vi "Resize Panel to Pane.vi"(8 "error in (no error)":errorcluster, 11 "ActorAutoRegPanel In":refnum<class "ActorAutoRegPanel.lvclass">) -> (0 "error out":errorcluster, 3 "ActorAutoRegPanel Out":refnum<class "ActorAutoRegPanel.lvclass">)   [LabVIEW 2015, in "TestViewables.lvlib" / "ActorAutoRegPanel.lvclass"]
doc: "<License>\nCopyright © 2017 Composed Systems, LLC | All rights reserved\nwww.composed.io\n\nAuthor: Ethan Stern <ethan.stern@composed.io>\n\nThis software is provided \"AS IS\" WITHOUT WARRANTIES, either express or implied, AND IS FOR EDUCATIONAL PURPOSES ONLY.\n</License>"
uses:
  ActorAutoRegPanel.lvclass
  DialogBox/OneButtonDialogBox/OneButtonDialogBox.lvclass
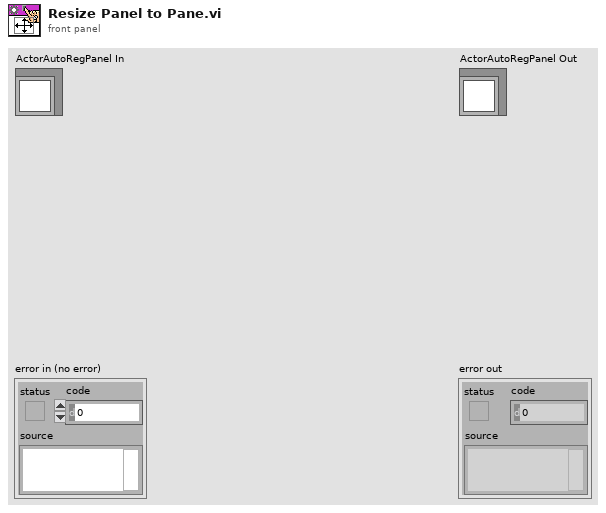
[diagram p1: front panel]
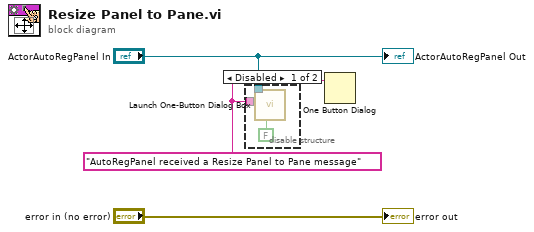
[diagram p0: block diagram]
diagram:
  w1 = "AutoRegPanel received a Resize Panel to Pane message" ("Message Text")
  n1 = disable-structure shown="Disabled" {
    disable-tunnel: "ActorAutoRegPanel In" -> [w6 _]
    disable-tunnel: w1 -> [w4 _]
    frame Disabled {
      n2 = call "Launch One-Button Dialog Box.vi"("Modal? (T)"=FALSE, "Message Text"=w4, "Dialog Launcher"=w6) -> ()  [unwired: 8 in, 1 out]
    }
    frame Enabled {
    }
  }
  n3 = One Button Dialog(message=w1) -> ()  [unwired: 1 in, 1 out]
  "error out" <- "error in (no error)"
  "ActorAutoRegPanel Out" <- "ActorAutoRegPanel In"
